vi "Configure Impedance.vi"(7 "Impedance":enum16{"50Ω", "1 MΩ"}(ring), 8 "error in (no error)":errorcluster, 11 "VISA resource name":refnum<visa-resource-name>) -> (0 "error out":errorcluster, 3 "VISA resource name out":refnum<visa-resource-name>)   [LabVIEW 2018, in "Fluke 9500B.lvlib"]
uses:
  <instrlib>/Fluke 9500B/Fluke 9500B.lvlib
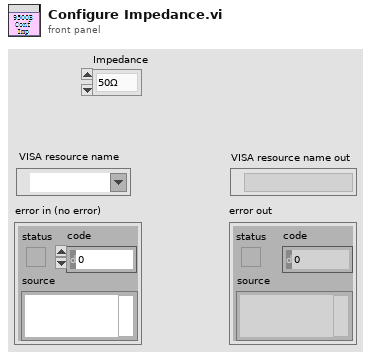
[diagram p1: front panel]
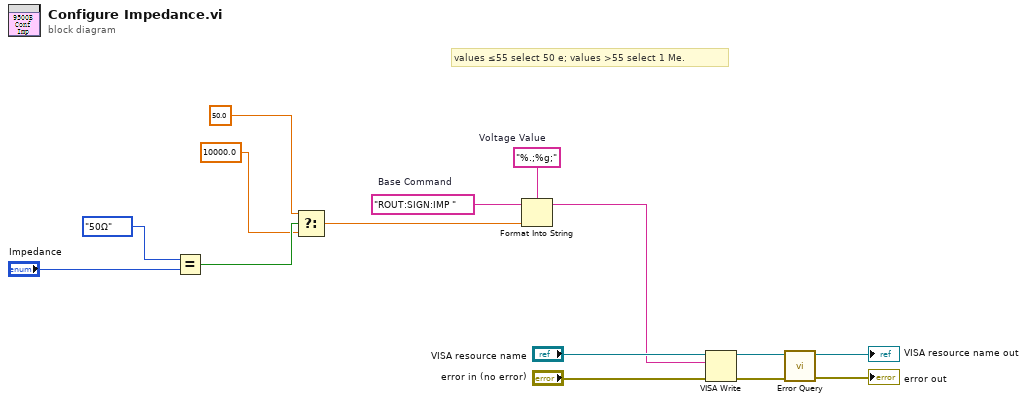
[diagram p0: block diagram]
diagram:
  w13 = "%.;%g;"  # Voltage Value
  w12 = "ROUT:SIGN:IMP "  # Base Command
  # "values ≤55 select 50 e; values >55 select 1 Me."
  n1 = Equal?(x=enum16{"50Ω", "1 MΩ"}."50Ω", y="Impedance") -> (x = y?=w8:bool)
  n2 = Select(t=50.0 ("输入 1"), s=w8, f=10000.0 ("输入 1")) -> (s? t:f=w5:dbl)
  n3 = Format Into String(format string=w13, initial string=w12, w5) -> (resulting string=w11:string)  [unwired: 1 in, 1 out]
  n4 = VISA Write(VISA resource name="VISA resource name", write buffer=w11, error in (no error)="error in (no error)") -> (VISA resource name out=w2:refnum<visa-resource-name>, error out=w1:errorcluster)  [unwired: 1 out]
  n5 = call <instrlib>:"Error Query.vi"("error in (no error)"=w1, "VISA resource name"=w2) -> ("error out"=→"error out":errorcluster, "VISA resource name out"=→"VISA resource name out":refnum<visa-resource-name>)  [unwired: 6 in, 2 out]
